vi "Register.vi"(10 "element (unused)":cluster{"cmd":string, "data":variant}, 11 "data in":refnum<class "EventMessengerData.lvclass">) -> (2 "event registration refnum":refnum<event-registration>, 3 "data out":refnum<class "EventMessengerData.lvclass">)   [LabVIEW 2019, in "Cmd-Data Event Messenger.lvlib" / "EventMessengerData.lvclass"]
uses:
  EventMessengerData.lvclass
  EventMessengerData.lvclass/EventMessengerData.ctl
  Event Data.ctl
  Cmd-Data Event Messenger.lvlib
panel:
  # "See note on block diagram."
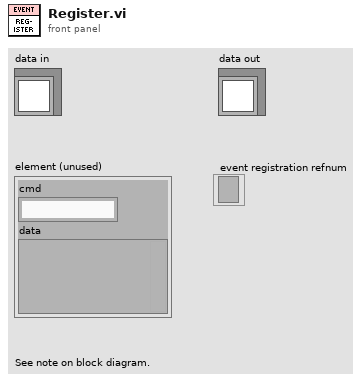
[diagram p1: front panel]
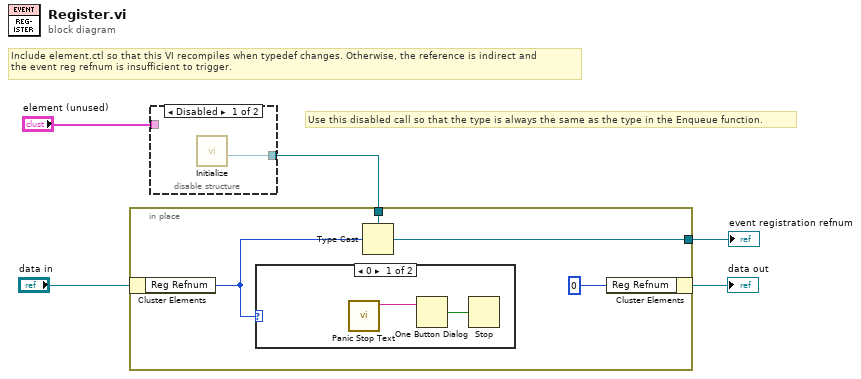
[diagram p0: block diagram]
diagram:
  # "Include element.ctl so that this VI recompiles when typedef changes. Otherwise, the reference is indirect and\nthe event reg refnum is insufficient to trigger."
  # "Use this disabled call so that the type is always the same as the type in the Enqueue function."
  n1 = disable-structure "Diagram Disable Structure" shown="Disabled" {
    disable-tunnel: [w6 _] -> w5
    disable-tunnel: "element (unused)" -> [_ _]
    frame Disabled {
      n2 = call "Initialize.vi"() -> ("Event Registration Refnum"=w6:refnum<event-registration>)  [unwired: 10 in, 1 out]
    }
    frame Enabled {
    }
  }
  n3 = in-place {
    in-place-border: w5 -> [w10]
    in-place-border: [w9] -> w1
    n4 = in-place-cluster #1("data in") -> ("Reg Refnum"=w7:u32)
    n5 = case shown="0" w7 {
      frame 0 {
        n6 = call "Panic Stop Text.vi"() -> ("Text"=w11:string)  [unwired: 11 in]
        n7 = One Button Dialog(message=w11) -> (true=w12:bool)  [unwired: 1 in]
        n8 = Stop(stop? (T)=w12) -> ()
      }
      frame Default {
      }
    }
    n9 = Type Cast(type=w10, x=w7) -> (*(type *) &x=w9:refnum<event-registration>)
    n10 = in-place-cluster #1("Reg Refnum"=u32 0) -> (→"data out":refnum<class "EventMessengerData.lvclass">)
  }
  "event registration refnum" <- w1
